vi "Read Reference Value.vi"(8 "error in (no error)":errorcluster, 11 "VISA resource name":refnum<visa-resource-name>) -> (0 "error out":errorcluster, 1 "Reference Unit":i32(ring) items=["No Result"=-1, "V"=0, "dBm"=1, "A"=2, "Ohm"=3, "Hz"=4], 2 "Reference Value":dbl, 3 "VISA resource name out":refnum<visa-resource-name>)   [LabVIEW 2012, in "Fluke 5080.lvlib"]
doc: "Returns the output reference values."
uses:
  <instrlib>/Fluke 5080/Fluke 5080.lvlib
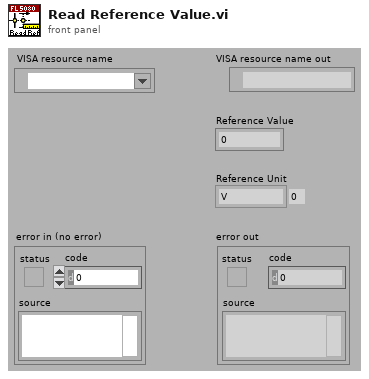
[diagram p1: front panel]
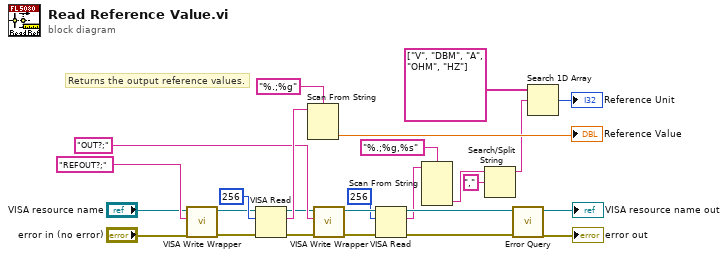
[diagram p0: block diagram]
diagram:
  # "Returns the output reference values."
  n1 = call <instrlib>:"VISA Write Wrapper.vi"("error in (no error)"="error in (no error)", "Write Buffer"="REFOUT?;", "VISA resource name"="VISA resource name") -> ("error out"=w19:errorcluster, "VISA resource name out"=w20:refnum<visa-resource-name>)  [unwired: 7 out]
  n2 = VISA Read(VISA resource name=w20, byte count=u32 256, error in (no error)=w19) -> (VISA resource name out=w14:refnum<visa-resource-name>, read buffer=w24:string, error out=w11:errorcluster)  [unwired: 1 out]
  n3 = Scan From String(format string="%.;%g", input string=w24) -> (output 1=→"Reference Value":dbl)  [unwired: 2 in, 4 out]
  n4 = call <instrlib>:"VISA Write Wrapper.vi"("error in (no error)"=w11, "Write Buffer"="OUT?;", "VISA resource name"=w14) -> ("error out"=w10:errorcluster, "VISA resource name out"=w13:refnum<visa-resource-name>)  [unwired: 7 out]
  n5 = VISA Read(VISA resource name=w13, byte count=u32 256, error in (no error)=w10) -> (VISA resource name out=w12:refnum<visa-resource-name>, read buffer=w7:string, error out=w9:errorcluster)  [unwired: 1 out]
  n6 = Scan From String(format string="%.;%g,%s", input string=w7) -> (output 2=w3:string)  [unwired: 2 in, 6 out]
  n7 = Search/Split String(string=w3, search string/char (-)=",") -> (substring before match=w1:string)  [unwired: 3 out]
  n8 = call <instrlib>:"Error Query.vi"("error in (no error)"=w9, "VISA resource name"=w12) -> ("error out"=→"error out":errorcluster, "VISA resource name out"=→"VISA resource name out":refnum<visa-resource-name>)  [unwired: 8 out]
  n9 = Search 1D Array(1D array=string[] ["V", "DBM", "A", "OHM", "HZ"], element=w1) -> (index of element=→"Reference Unit":i32)  [unwired: 1 out]
